vi "Read session reservation.vi"(8 "error in (no error)":errorcluster, 11 "Abstract_Instrument in":refnum<class "Abstract_Instrument.lvclass">) -> (0 "error out":errorcluster, 2 "MeasurementLink Session Management V1.lvlib:Session Reservation.lvclass":refnum<class "Session Reservation.lvclass">, 3 "Abstract_Instrument out":refnum<class "Abstract_Instrument.lvclass">)   [LabVIEW 2021, in "Abstract_Instrument.lvclass"]
uses:
  Abstract_Instrument.lvclass
  <vilib>/MeasurementLink/MeasurementLink Session Management V1/Session Reservation/Session Reservation.lvclass
  Abstract_Instrument.lvclass/Abstract_Instrument.ctl
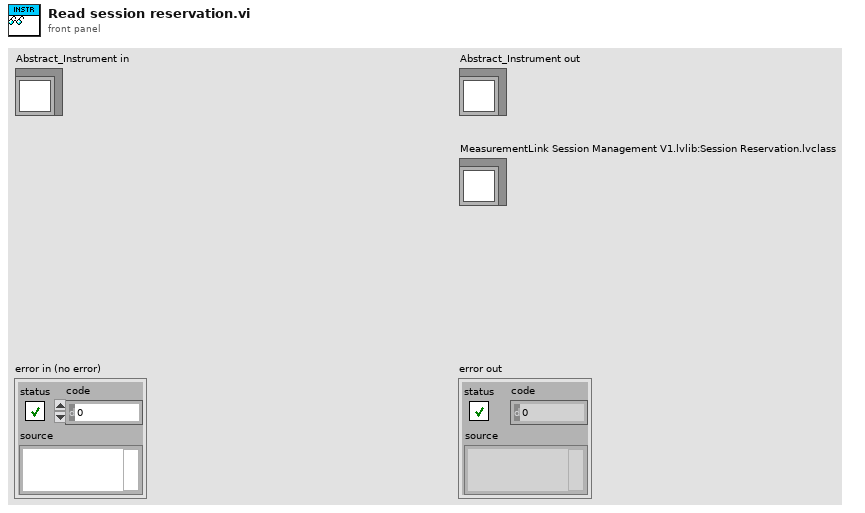
[diagram p1: front panel]
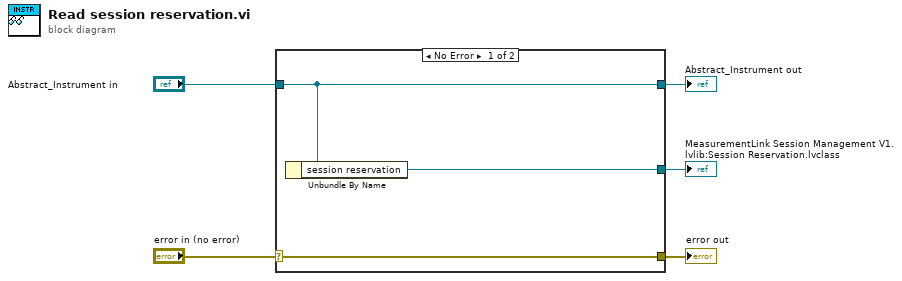
[diagram p0: block diagram]
diagram:
  n1 = case shown="No Error" "error in (no error)" {
    selector: "error in (no error)" -> [w8 w9]
    tunnel: [w8 w9] -> w4
    tunnel: [w7 w10] -> w2
    tunnel: "Abstract_Instrument in" -> [w7 w10]
    tunnel: [w6 _] -> w1
    frame No Error {
      n2 = Unbundle By Name(w7) -> ("session reservation"=w6:refnum<class "Session Reservation.lvclass">)
    }
    frame Error {
    }
  }
  "error out" <- w4
  "Abstract_Instrument out" <- w2
  "MeasurementLink Session Management V1.lvlib:Session Reservation.lvclass" <- w1
